vi "refmgr_get.vi"   [LabVIEW 2014, in "RefManager(dev).lvlib"]
uses:
  RefManager(dev).lvlib
  <userlib>/_NEVSTOP/TagDB/Core/tagDB_Def.ctl
  <userlib>/_NEVSTOP/TagDB/Core/TagDB.lvlib
  _Support/XNode/refmgr_get.xnode/refmgr_get.xnode
  <userlib>/_NEVSTOP/TagDB/Core/_Support/Properties/tagDB dbChanged.vi
  <userlib>/_NEVSTOP/TagDB/Core/_Support/Properties/tagDB getTags.vi
  <userlib>/_NEVSTOP/TagDB/Core/_Support/Access/_variant.vi
  <userlib>/_NEVSTOP/TagDB/Core/_Support/Error/_Clear Errors.vi
  <userlib>/_NEVSTOP/TagDB/Core/_XNode/tagDB_value.xnode/tagDB_value.xnode
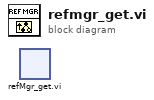
[diagram p0: block diagram]
diagram:
  n1 = xnode "refMgr_get.vi"() -> ()  [unwired: 4 in, 4 out]
